vi "9068-Temp-scan-engine.vi"(3 "MessageFormat":string, 5 "error in (no error)":errorcluster) -> (15 "updated?":bool[](array[boolean]), 16 "Messages":string[](array[string]), 19 "error out":errorcluster)   [LabVIEW 2024]
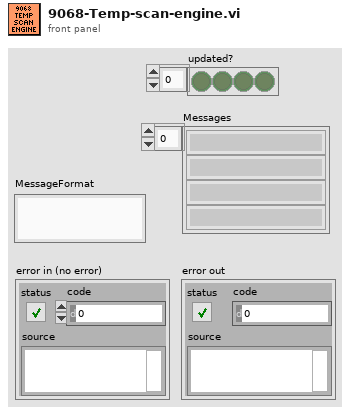
[diagram p1: front panel]
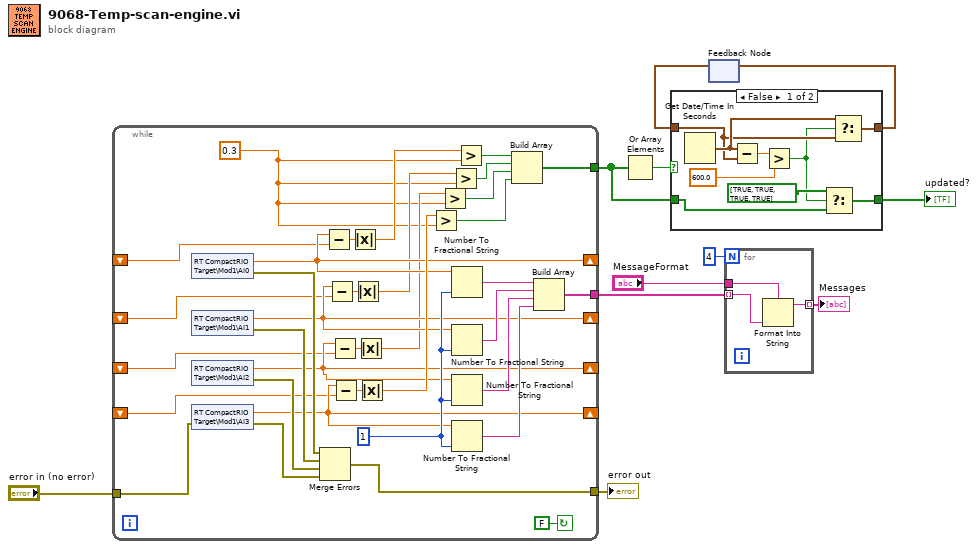
[diagram p0: block diagram]
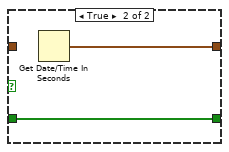
[diagram p2: hidden frame]
diagram:
  n1 = while {
    shift-right: [w19] -> _
    shift-left: _ -> [w16]
    tunnel: "error in (no error)" -> [w40]
    tunnel: [w39] -> w10
    shift-right: [w20] -> _
    shift-left: _ -> [w17]
    shift-right: [w21] -> _
    shift-left: _ -> [w18]
    shift-right: [w32] -> _
    shift-left: _ -> [w31]
    tunnel: [w38] -> w2
    tunnel: [w33] -> w9
    stop <- FALSE continue-if-true
    w12 = 0.3 ("y")
    w42 = i16 1 ("precision (6)")
    n2 = shared-variable "RT CompactRIO Target\\Mod1\\AI0"() -> (w19:dbl, error out=w43:errorcluster)  [unwired: 1 in]
    n3 = shared-variable "RT CompactRIO Target\\Mod1\\AI1"() -> (w20:dbl, error out=w44:errorcluster)  [unwired: 1 in]
    n4 = shared-variable "RT CompactRIO Target\\Mod1\\AI2"() -> (w21:dbl, error out=w45:errorcluster)  [unwired: 1 in]
    n5 = shared-variable "RT CompactRIO Target\\Mod1\\AI3"(error in=w40) -> (w32:dbl, error out=w46:errorcluster)
    n6 = Merge Errors(w43, w44, w45, w46) -> (w39:errorcluster)
    n7 = Subtract(x=w19, y=w16) -> (x-y=w22:dbl)
    n8 = Subtract(x=w20, y=w17) -> (x-y=w23:dbl)
    n9 = Subtract(x=w21, y=w18) -> (x-y=w24:dbl)
    n10 = Subtract(x=w32, y=w31) -> (x-y=w30:dbl)
    n11 = Absolute Value(x=w22) -> (abs(x)=w13:dbl)
    n12 = Absolute Value(x=w23) -> (abs(x)=w15:dbl)
    n13 = Absolute Value(x=w24) -> (abs(x)=w14:dbl)
    n14 = Absolute Value(x=w30) -> (abs(x)=w29:dbl)
    n15 = Greater?(x=w29, y=w12) -> (0:w28:bool)
    n16 = Greater?(x=w14, y=w12) -> (0:w27:bool)
    n17 = Greater?(x=w15, y=w12) -> (0:w26:bool)
    n18 = Number To Fractional String(number=w19, precision (6)=w42) -> (F-format string=w37:string)  [unwired: 2 in]
    n19 = Number To Fractional String(number=w20, precision (6)=w42) -> (F-format string=w36:string)  [unwired: 2 in]
    n20 = Number To Fractional String(number=w21, precision (6)=w42) -> (F-format string=w35:string)  [unwired: 2 in]
    n21 = Number To Fractional String(number=w32, precision (6)=w42) -> (F-format string=w34:string)  [unwired: 2 in]
    n22 = Greater?(x=w13, y=w12) -> (0:w25:bool)
    n23 = Build Array(w25, w26, w27, w28) -> (w38:bool[])
    n24 = Build Array(w37, w36, w35, w34) -> (w33:string[])
  }
  "error out" <- w10
  n25 = Or Array Elements(Boolean array=w2) -> (logical OR=w5:bool)
  n26 = feedback #1() -> (w3:timestamp)  [unwired: 1 in]
  n27 = case shown="False" w5 {
    tunnel: [w49 w57] -> w4
    tunnel: w3 -> [w48 _]
    tunnel: w2 -> [w53 w56]
    tunnel: [w51 w56] -> w1
    frame False {
      n28 = Get Date/Time In Seconds() -> (seconds since 1Jan1904=w50:timestamp)
      n29 = Subtract(x=w50, y=w48) -> (x-y=w55:dbl)
      n30 = Greater?(x=w55, y=600.0) -> (0:w47:bool)
      n31 = Select(t=bool[] [TRUE, TRUE, TRUE, TRUE], s=w47, f=w53) -> (s? t:f=w51:bool[])
      n32 = Select(t=w50, s=w47, f=w48) -> (s? t:f=w49:timestamp)
    }
    frame True {
      n33 = Get Date/Time In Seconds() -> (seconds since 1Jan1904=w57:timestamp)
    }
  }
  "updated?" <- w1
  n34 = feedback-in #1(w4) -> ()
  n35 = for {
    N: 4 -> [_]
    tunnel: w9 -> [w58] mode=indexing
    tunnel: "MessageFormat" -> [w60]
    tunnel: [w59] -> w6 mode=indexing
    n36 = Format Into String(format string=w60, w58) -> (resulting string=w59:string)  [unwired: 2 in, 1 out]
  }
  "Messages" <- w6
